vi "Insert Child Attributes.vi"(10 "Child Attributes":refnum<class "Attributes.lvclass">, 11 "Core Actor in":refnum<class "Core Actor.lvclass">) -> (3 "Core Actor out":refnum<class "Core Actor.lvclass">)   [LabVIEW 2025, in "jettl.lvlib" / "Core Actor.lvlib" / "Core Actor.lvclass"]
uses:
  Core Actor.lvclass
  Attributes/Attributes.lvclass
  Core Actor.lvclass/Core Actor.ctl
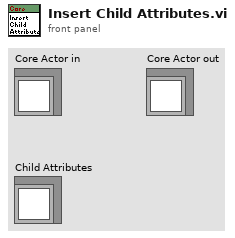
[diagram p1: front panel]
types:
  T1 = typedef "jettl.lvlib/Core Actor.lvlib/Core Actor.lvclass/Child Attributes Map.ctl" = map{string, refnum<class "Attributes.lvclass">}
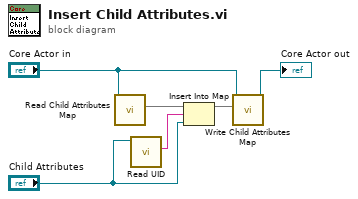
[diagram p0: block diagram]
diagram:
  n1 = call "Read Child Attributes Map.vi"("Core Actor in"="Core Actor in") -> ("Child Attributes Map"=w2:T1)  [unwired: 10 in]
  n2 = call-dynamic "Read UID.vi"("Attributes in"="Child Attributes") -> ("UID"=w3:string)  [unwired: 10 in]
  n3 = Insert Into Map(map in=w2, key=w3, value="Child Attributes") -> (map out=w1:T1)  [unwired: 2 out]
  n4 = call "Write Child Attributes Map.vi"("Child Attributes Map"=w1, "Core Actor in"="Core Actor in") -> ("Core Actor out"=→"Core Actor out":refnum<class "Core Actor.lvclass">)  [unwired: 9 in]
